vi "Merenje_1_ACC.vi"() -> ()   [LabVIEW 2016]
uses:
  <vilib>/Waveform/WDTOps.llb/WDT Index Channel DBL.vi
panel:
  out "ACC 3":dynamicdata(graph)
  out "ACC 2":dynamicdata(graph)
  out "ACC 1":dynamicdata(graph)
  in  "stop (F)":bool
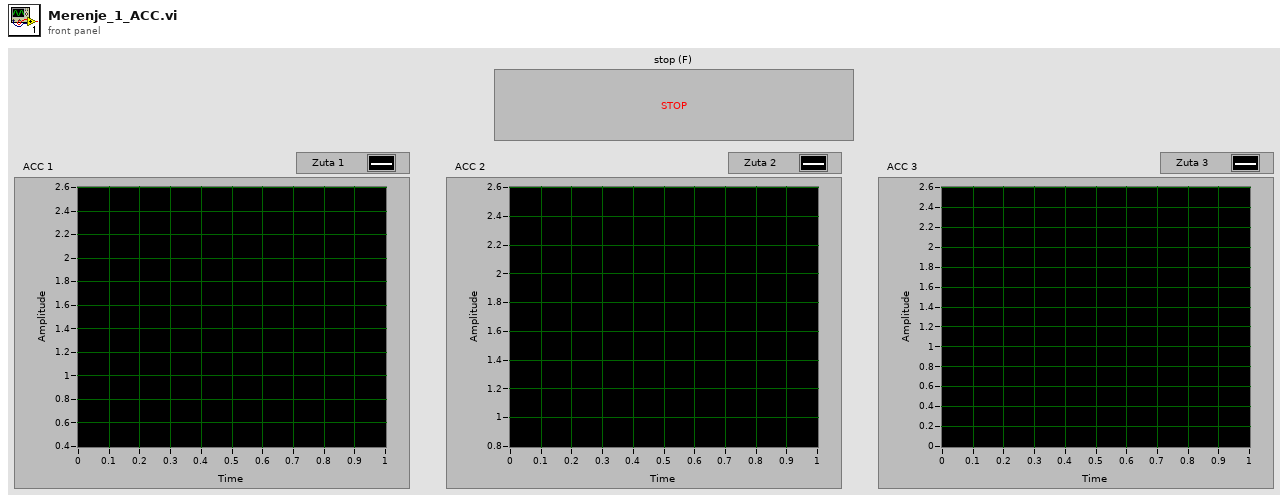
[diagram p1: front panel]
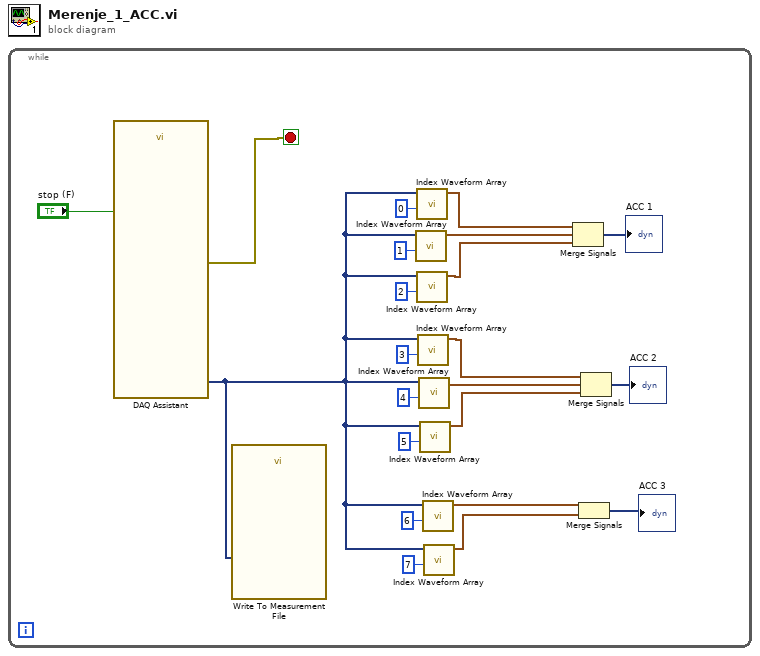
[diagram p0: block diagram]
diagram:
  n1 = while {
    stop <- w2 stop-if-true
    n2 = call "DAQ Assistant"("stop (F)"="stop (F)") -> ("data"=w1:dynamicdata, "error out"=w2:errorcluster)  [unwired: 15 in, 2 out]
    n3 = call "Write To Measurement File"("Signals"=w1) -> ()  [unwired: 16 in, 3 out]
    n4 = call-poly <vilib>:"Index Waveform Array.vi"("index"=1, "waveform array"=w1) -> ("waveform"=w8:waveform(dbl))  [unwired: 8 in, 1 out]
    n5 = call-poly <vilib>:"Index Waveform Array.vi"("index"=0, "waveform array"=w1) -> ("waveform"=w7:waveform(dbl))  [unwired: 8 in, 1 out]
    n6 = call-poly <vilib>:"Index Waveform Array.vi"("index"=2, "waveform array"=w1) -> ("waveform"=w6:waveform(dbl))  [unwired: 8 in, 1 out]
    n7 = call-poly <vilib>:"Index Waveform Array.vi"("index"=3, "waveform array"=w1) -> ("waveform"=w11:waveform(dbl))  [unwired: 8 in, 1 out]
    n8 = call-poly <vilib>:"Index Waveform Array.vi"("index"=4, "waveform array"=w1) -> ("waveform"=w12:waveform(dbl))  [unwired: 8 in, 1 out]
    n9 = call-poly <vilib>:"Index Waveform Array.vi"("index"=5, "waveform array"=w1) -> ("waveform"=w10:waveform(dbl))  [unwired: 8 in, 1 out]
    n10 = call-poly <vilib>:"Index Waveform Array.vi"("index"=6, "waveform array"=w1) -> ("waveform"=w5:waveform(dbl))  [unwired: 8 in, 1 out]
    n11 = call-poly <vilib>:"Index Waveform Array.vi"("index"=7, "waveform array"=w1) -> ("waveform"=w4:waveform(dbl))  [unwired: 8 in, 1 out]
    n12 = Merge Signals(w7, w8, w6) -> (→"ACC 1":dynamicdata)
    n13 = Merge Signals(w5, w4) -> (→"ACC 3":dynamicdata)
    n14 = Merge Signals(w11, w12, w10) -> (→"ACC 2":dynamicdata)
  }
